vi "Set Translation and Rotation.vi"(0 "SceneObject in":refnum<vi>, 1 "Transformation.GetTranslation in":T1, 2 "X axis deg":sgl(slide) min=0 max=360 step=1 scale=0.0..360.0, 3 "Y axis deg":sgl(slide) min=0 max=360 step=1 scale=0.0..360.0, 4 "Z axis deg":sgl(slide) min=0 max=360 step=1 scale=0.0..360.0, 7 "Initial Rotation Axis":T1, 9 "Initial Rotation Angle":sgl, 11 "Relative?":bool) -> (14 "SceneObject out":refnum<vi>, 16 "Transformation.GetTranslation out":T1, 17 "Rotation Axis Out":T1, 18 "Angle Out":sgl)   [LabVIEW 2021]
uses:
  <vilib>/Utility/miscctls.llb/LV3DPointTypeDef.ctl
  <vilib>/picture/3D Picture Control/NI_3D Picture Control.lvlib
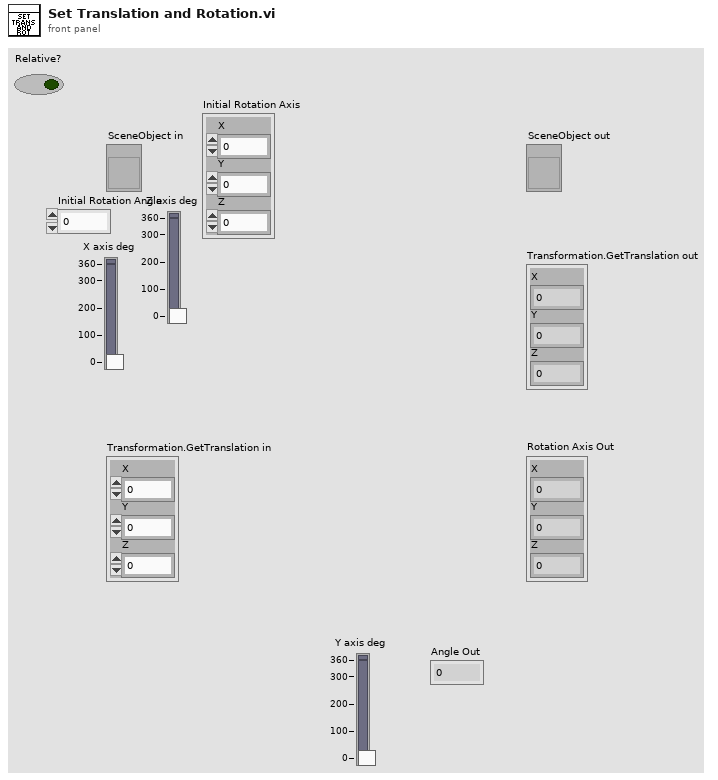
[diagram p1: front panel]
types:
  T1 = typedef "LV3DPointTypeDef.ctl" = cluster{"X":sgl, "Y":sgl, "Z":sgl}
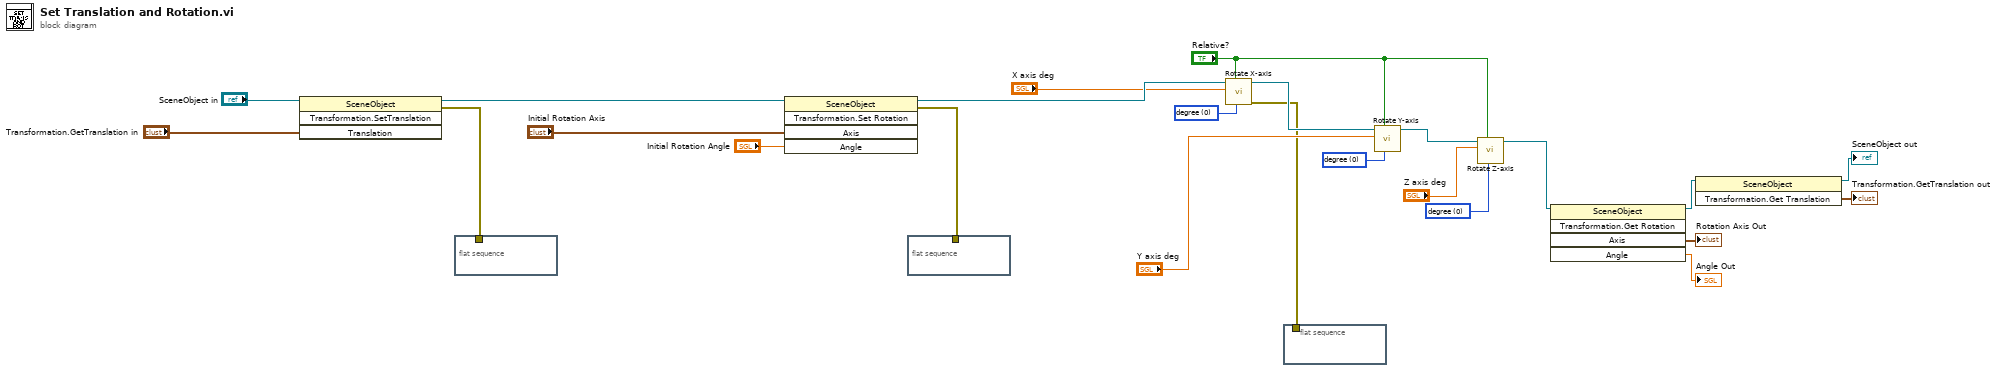
[diagram p0: block diagram]
diagram:
  w6 = u16 0 items=["degree", "radians"] ("angle unit")
  w11 = u16 0 items=["degree", "radians"] ("angle unit")
  w14 = u16 0 items=["degree", "radians"] ("angle unit")
  n1 = invoke class="SceneObject" method="Transformation.SetTranslation"(reference="SceneObject in", "Translation"="Transformation.GetTranslation in") -> (reference out=w18:refnum<vi>, error out=w3:errorcluster)  [unwired: 2 in, 2 out]
  n2 = flat-sequence {
    tunnel: w3 -> [_]
    frame #0 {
    }
  }
  n3 = invoke class="SceneObject" method="Transformation.Set Rotation"(reference=w18, "Axis"="Initial Rotation Axis", "Angle"="Initial Rotation Angle") -> (reference out=w16:refnum<vi>, error out=w2:errorcluster)  [unwired: 2 in, 3 out]
  n4 = flat-sequence {
    tunnel: w2 -> [_]
    frame #0 {
    }
  }
  n5 = call <vilib>:"Rotate X-axis.vi"("angle unit"=w14, "Relative?"="Relative?", "angle"="X axis deg", "Scene Object In"=w16) -> ("error out"=w1:errorcluster, "Scene Object Out"=w13:refnum<vi>)  [unwired: 6 in]
  n6 = flat-sequence {
    tunnel: w1 -> [_]
    frame #0 {
    }
  }
  n7 = call <vilib>:"Rotate Y-axis.vi"("angle unit"=w11, "Relative?"="Relative?", "angle"="Y axis deg", "Scene Object In"=w13) -> ("Scene Object Out"=w10:refnum<vi>)  [unwired: 6 in, 1 out]
  n8 = call <vilib>:"Rotate Z-axis.vi"("angle unit"=w6, "Relative?"="Relative?", "angle"="Z axis deg", "Scene Object In"=w10) -> ("Scene Object Out"=w9:refnum<vi>)  [unwired: 6 in, 1 out]
  n9 = invoke class="SceneObject" method="Transformation.Get Rotation"(reference=w9) -> (reference out=w22:refnum<vi>, "Axis"=→"Rotation Axis Out":T1, "Angle"=→"Angle Out":sgl)  [unwired: 4 in, 2 out]
  n10 = invoke class="SceneObject" method="Transformation.Get Translation"(reference=w22) -> (reference out=→"SceneObject out":refnum<vi>, "Transformation.GetTranslation"=→"Transformation.GetTranslation out":T1)  [unwired: 2 in, 1 out]
